vi "Generate Controller Event.vi"(8 "Error In":errorcluster, 10 "Event":refnum<class "Event.lvclass">, 11 "Controller In":refnum<class "Controller.lvclass">) -> (0 "Error Out":errorcluster, 3 "Controller Out":refnum<class "Controller.lvclass">)   [LabVIEW 2023, in "MVC Actors.lvlib" / "Controller.lvclass"]
doc: "This method generates/fires the Event wired to the input. Firing an event looks up all actors who Registered to listen to this Event and sends to them this Event on a Zero Coupling based message defined during Registration. Errors on broadcasting the event i.e. enqueuer of the registrant not existing, are ignored.\n\n<b>IMPORTANT</b> - Only call this method within actor core of your Controller Actor. From helper loops call the Send Generate Event message to self. This is to make sure your actor works with all registered listeners."
uses:
  Controller.lvclass
  Event/Event.lvclass
  Controller.lvclass/Controller.ctl
  Event Handler Details.ctl
  Event Handlers/Abstract Event Message for View/Abstract Event Message for View.lvclass
  C:/Program Files/National Instruments/LabVIEW 2023/vi.lib/ActorFramework/Message/Message.lvclass
  <vilib>/ActorFramework/Message Enqueuer/Message Enqueuer.lvclass
  Event Handlers/Abstract Event Message for View/Abstract Event Message for View.lvclass/Abstract Event Message for View.ctl
  <vilib>/ActorFramework/Message Enqueuer/Message Enqueuer.lvclass/Message Enqueuer.ctl
  Event Handlers/Abstract Event Message for View/Send Abstract Event Message for View.vi
  <vilib>/Utility/error.llb/Clear Errors.vi
  <vilib>/ActorFramework/Message Enqueuer/Enqueue.vi
  <vilib>/Utility/LVClass/Get LV Class Name.vi
  <resource>/AFDebug/Generate Trace for Message.vi
  <vilib>/ActorFramework/Message Priority Queue/Priority Enqueue.vi
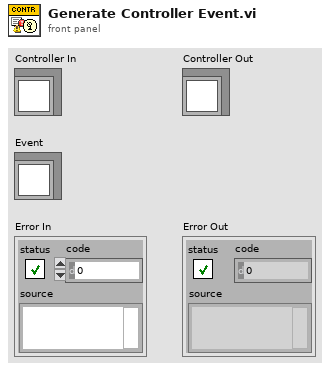
[diagram p1: front panel]
types:
  T1 = typedef "MVC Actors.lvlib/Controller.lvclass/Event Handler Details.ctl" = cluster{"Exclude From Broadcast":bool, "Paused":bool, "View Event Fire Handler":refnum<class "Abstract Event Message for View.lvclass">}
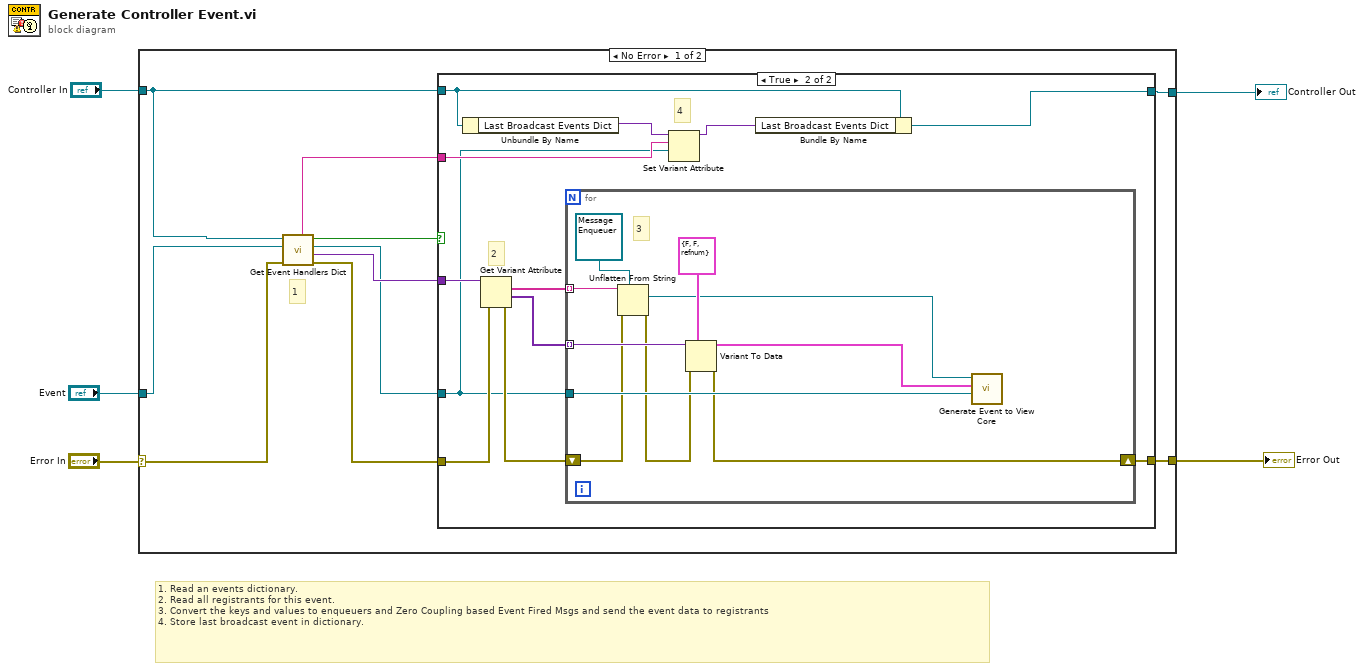
[diagram p0: block diagram]
diagram:
  # "1. Read an events dictionary.\n2. Read all registrants for this event.\n3. Convert the keys and values to enqueuers and Zero Coupling based Event Fired Msgs and send the event data to registrants\n4. Store last broadcast event in dictionary."
  n1 = case shown="No Error" "Error In" {
    selector: "Error In" -> [w11 w41]
    tunnel: "Controller In" -> [w8 w40]
    tunnel: "Event" -> [w10 _]
    tunnel: [w15 w41] -> w3
    tunnel: [w7 w40] -> w1
    frame No Error {
      # "1"
      n2 = call "Get Event Handlers Dict.vi"("error in (no error)"=w11, "Event In"=w10, "Controller in"=w8) -> ("error out"=w14:errorcluster, "Event Handlers Dict"=w13:variant, "Event out"=w9:refnum<class "Event.lvclass">, "Event Found"=w12:bool, "Event ID"=w6:string)  [unwired: 4 in]
      n3 = case shown="True" w12 {
        tunnel: w13 -> [_ w28]
        tunnel: w9 -> [_ w18]
        tunnel: w14 -> [w17 w25]
        tunnel: [w17 w29] -> w15
        tunnel: w8 -> [w16 w21]
        tunnel: [w16 w20] -> w7
        tunnel: w6 -> [_ w19]
        frame False {
        }
        frame True {
          # "4"
          # "2"
          n4 = Unbundle By Name(w21) -> ("Last Broadcast Events Dict"=w22:variant)
          n5 = Get Variant Attribute(Variant=w28, error in=w25) -> (names=w27:string[], values=w26:variant[], error out=w24:errorcluster)  [unwired: 2 in, 1 out]
          n6 = for {
            tunnel: w27 -> [w31] mode=indexing
            tunnel: w26 -> [w39] mode=indexing
            tunnel: w18 -> [w37]
            shift-right: [w30] -> w29
            shift-left: w24 -> [w36]
            # "3"
            n7 = Unflatten From String(type=refnum<class "Message Enqueuer.lvclass"> refnum ("Message Enqueuer"), binary string=w31, error in (no error)=w36) -> (value=w32:refnum<class "Message Enqueuer.lvclass">, error out=w35:errorcluster)  [unwired: 2 in, 1 out]
            n8 = Variant To Data(error in=w35, type=T1 {"Exclude From Broadcast"=FALSE, "Paused"=FALSE, "View Event Fire Handler"=refnum} ("Message Type"), Variant=w39) -> (data=w38:T1, error out=w30:errorcluster)
            n9 = call "Generate Event to View Core.vi"("Event in"=w37, "Event Handler Details"=w38, "Message Enqueuer in"=w32) -> ()  [unwired: 9 in]
          }
          n10 = Set Variant Attribute(Variant=w22, name=w19, value=w18) -> (Variant out=w23:variant)  [unwired: 1 in, 2 out]
          n11 = Bundle By Name(cluster=w21, "Last Broadcast Events Dict"=w23) -> (w20:refnum<class "Controller.lvclass">)
        }
      }
    }
    frame Error {
    }
  }
  "Error Out" <- w3
  "Controller Out" <- w1
